vi "Wait (with error terminals).vi"(8 "error in (no error)":errorcluster, 11 "milliseconds to wait":u32) -> (0 "error out":errorcluster, 3 "millisecond timer value":u32)   [LabVIEW 2014, in "COSYLib.lvlib"]
doc: "Exactly the same as the \"Wait\" function in LabVIEW, but with error terminals. This allows for using data flow to specify sequences.\nNOTE: does *not* wait if there's an error on the \"error in\" terminal."
uses:
  COSYLib.lvlib
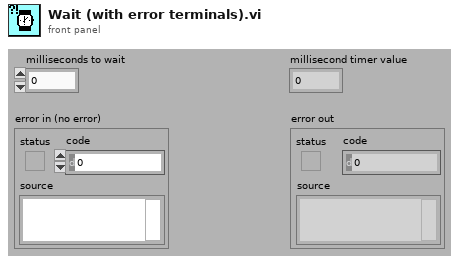
[diagram p1: front panel]
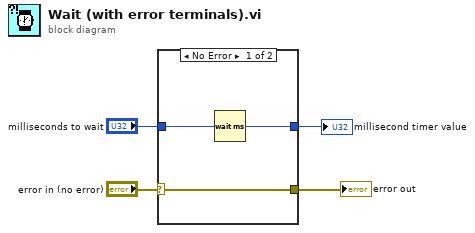
[diagram p0: block diagram]
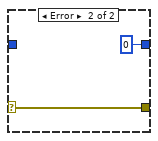
[diagram p2: hidden frame]
diagram:
  n1 = case shown="No Error" "error in (no error)" {
    selector: "error in (no error)" -> [w5 w9]
    tunnel: "milliseconds to wait" -> [w7 _]
    tunnel: [w6 u32 0 ("millisecond timer value")] -> w3
    tunnel: [w5 w9] -> w1
    frame No Error {
      n2 = Wait (ms)(milliseconds to wait=w7) -> (millisecond timer value=w6:u32)
    }
    frame Error {
    }
  }
  "millisecond timer value" <- w3
  "error out" <- w1
